vi "smartmeshIP mesh health.vi"(5 "mote and link status":T5, 11 "error in":errorcluster, 12 "mac adresses":T2) -> (2 "waveform output cluster":T1, 4 "Mote Status":T4(array[cluster]) {"mote state" items=["Lost"=0, "Negotiating"=1, "Operational"=4]}, 6 "Primary link status":T3(array[cluster]), 10 "last packet type dust":i32[](array[numeric]), 14 "Online":bool[](array[boolean]), 15 "error out":errorcluster)   [LabVIEW 2017]
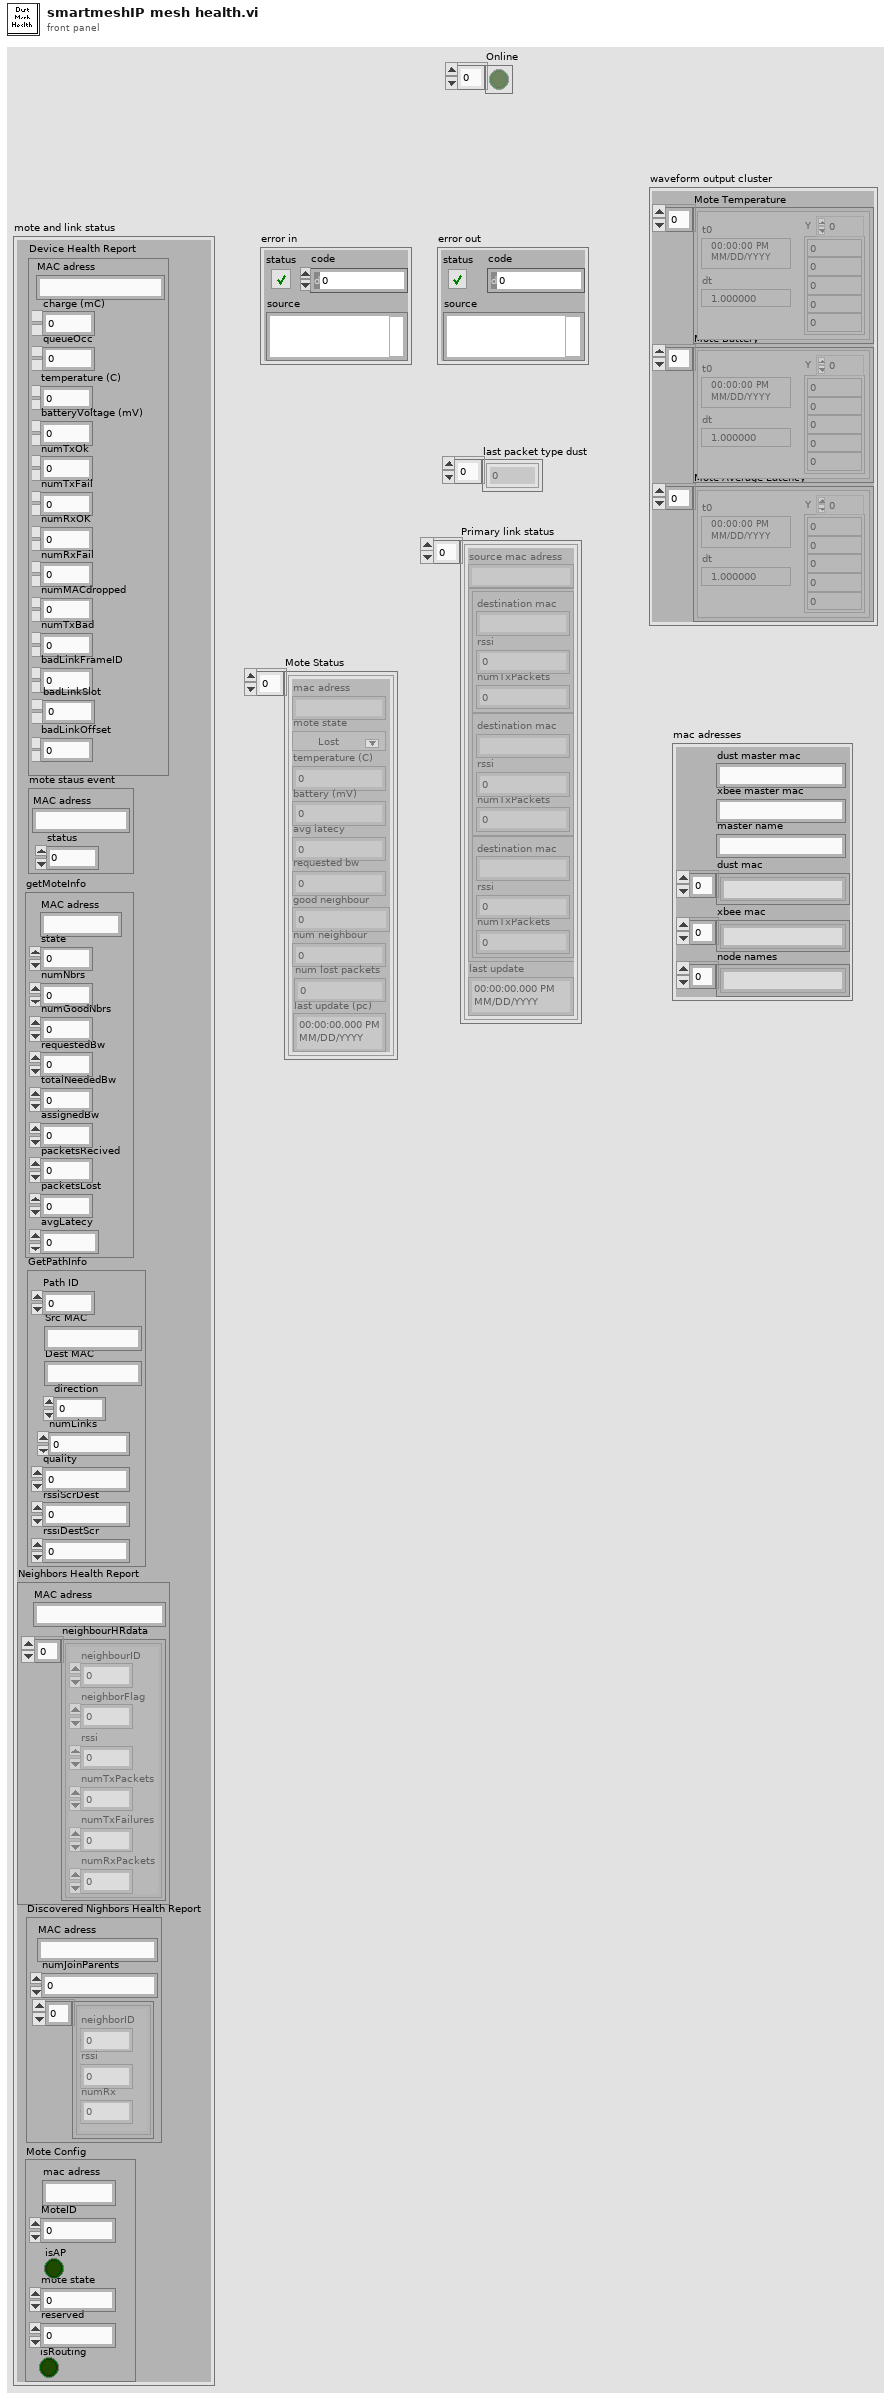
[diagram p1: front panel]
types:
  T1 = cluster{"Mote Temperature":waveform(i32)[], "Mote Battery":waveform(i32)[], "Mote Average Latency":waveform(i32)[]}
  T2 = cluster{"dust master mac":string, "xbee master mac":string, "master name":string, "dust mac":string[], "xbee mac":string[], "node names":string[]}
  T3 = cluster{"source mac adress":string, cluster{"destination mac":string, "rssi":i8, "numTxPackets":u16}[], "last update":timestamp}[]
  T4 = cluster{"mac adress":string, "mote state":u8, "temperature (C)":i8, "battery (mV)":u16, "avg latecy":u32, "requested bw":u32, "good neighbour":u8, "num neighbour":u8, "num lost packets":u8, "last update (pc)":timestamp}[]
  T5 = cluster{"Device Health Report":cluster{"MAC adress":string, "charge (mC)":u32, "queueOcc":u8, "temperature (C)":i8, "batteryVoltage (mV)":u16, "numTxOk":u16, "numTxFail":u16, "numRxOK":u16, "numRxFail":u16, "numMACdropped":u8, "numTxBad":u8, "badLinkFrameID":u8, "badLinkSlot":u32, "badLinkOffset":u8}, "mote staus event":cluster{"MAC adress":string, "status":u8}, "getMoteInfo":cluster{"MAC adress":string, "state":u8, "numNbrs":u8, "numGoodNbrs":u8, "requestedBw":u32, "totalNeededBw":u32, "assignedBw":u32, "packetsRecived":u32, "packetsLost":u32, "avgLatecy":u32}, "GetPathInfo":cluster{"Path ID":u8, "Src MAC":string, "Dest MAC":string, "direction":u8, "numLinks":u8, "quality":u8, "rssiScrDest":i8, "rssiDestScr":i8}, "Neighbors Health Report":cluster{"MAC adress":string, "neighbourHRdata":cluster{"neighbourID":u16, "neighborFlag":u8, "rssi":i8, "numTxPackets":u16, "numTxFailures":u16, "numRxPackets":u16}[]}, "Discovered Nighbors Health Report":cluster{"MAC adress":string, "numJoinParents":u8, cluster{"neighborID":u16, "rssi":i8, "numRx":u8}[]}, "Mote Config":cluster{"mac adress":string, "MoteID":u16, "isAP":bool, "mote state":u8, "reserved":u8, "isRouting":bool}}
  T6 = cluster{"MAC adress":string, "charge (mC)":u32, "queueOcc":u8, "temperature (C)":i8, "batteryVoltage (mV)":u16, "numTxOk":u16, "numTxFail":u16, "numRxOK":u16, "numRxFail":u16, "numMACdropped":u8, "numTxBad":u8, "badLinkFrameID":u8, "badLinkSlot":u32, "badLinkOffset":u8}
  T7 = cluster{"MAC adress":string, "neighbourHRdata":cluster{"neighbourID":u16, "neighborFlag":u8, "rssi":i8, "numTxPackets":u16, "numTxFailures":u16, "numRxPackets":u16}[]}
  T8 = cluster{"MAC adress":string, "state":u8, "numNbrs":u8, "numGoodNbrs":u8, "requestedBw":u32, "totalNeededBw":u32, "assignedBw":u32, "packetsRecived":u32, "packetsLost":u32, "avgLatecy":u32}
  T9 = cluster{"mac adress":string, "MoteID":u16, "isAP":bool, "mote state":u8, "reserved":u8, "isRouting":bool}
  T10 = cluster{"mac adress":string, "rssi":u8, "numTxPackets":i8}
  T11 = cluster{"time string 2":string, "mote state":u8, "temperature (C)":i8, "state":u16, "avgLatecy":u32, "avgLatecy 2":u32, "numTxBad":u8, "numTxBad 2":u8, "numTxBad 3":u8, "time string":timestamp}
  T12 = cluster{"mac adress":string, "rssi":u8, "numTxPackets":i8}[][]
  T13 = cluster{"time string 2":string, "mote state":u8, "temperature (C)":i8, "state":u16, "avgLatecy":u32, "avgLatecy 2":u32, "numTxBad":u8, "numTxBad 2":u8, "numTxBad 3":u8, "time string":timestamp}[]
  T14 = cluster{"neighbourID":u16, "neighborFlag":u8, "rssi":i8, "numTxPackets":u16, "numTxFailures":u16, "numRxPackets":u16}[]
  T15 = cluster{"mac adress":string, cluster{"Dest MAC":string, "rssi":u8, "numTxPackets":u16}[], "seconds since 1Jan1904":timestamp}
  T16 = cluster{waveform(i32)[], waveform(i32)[], waveform(i32)[]}
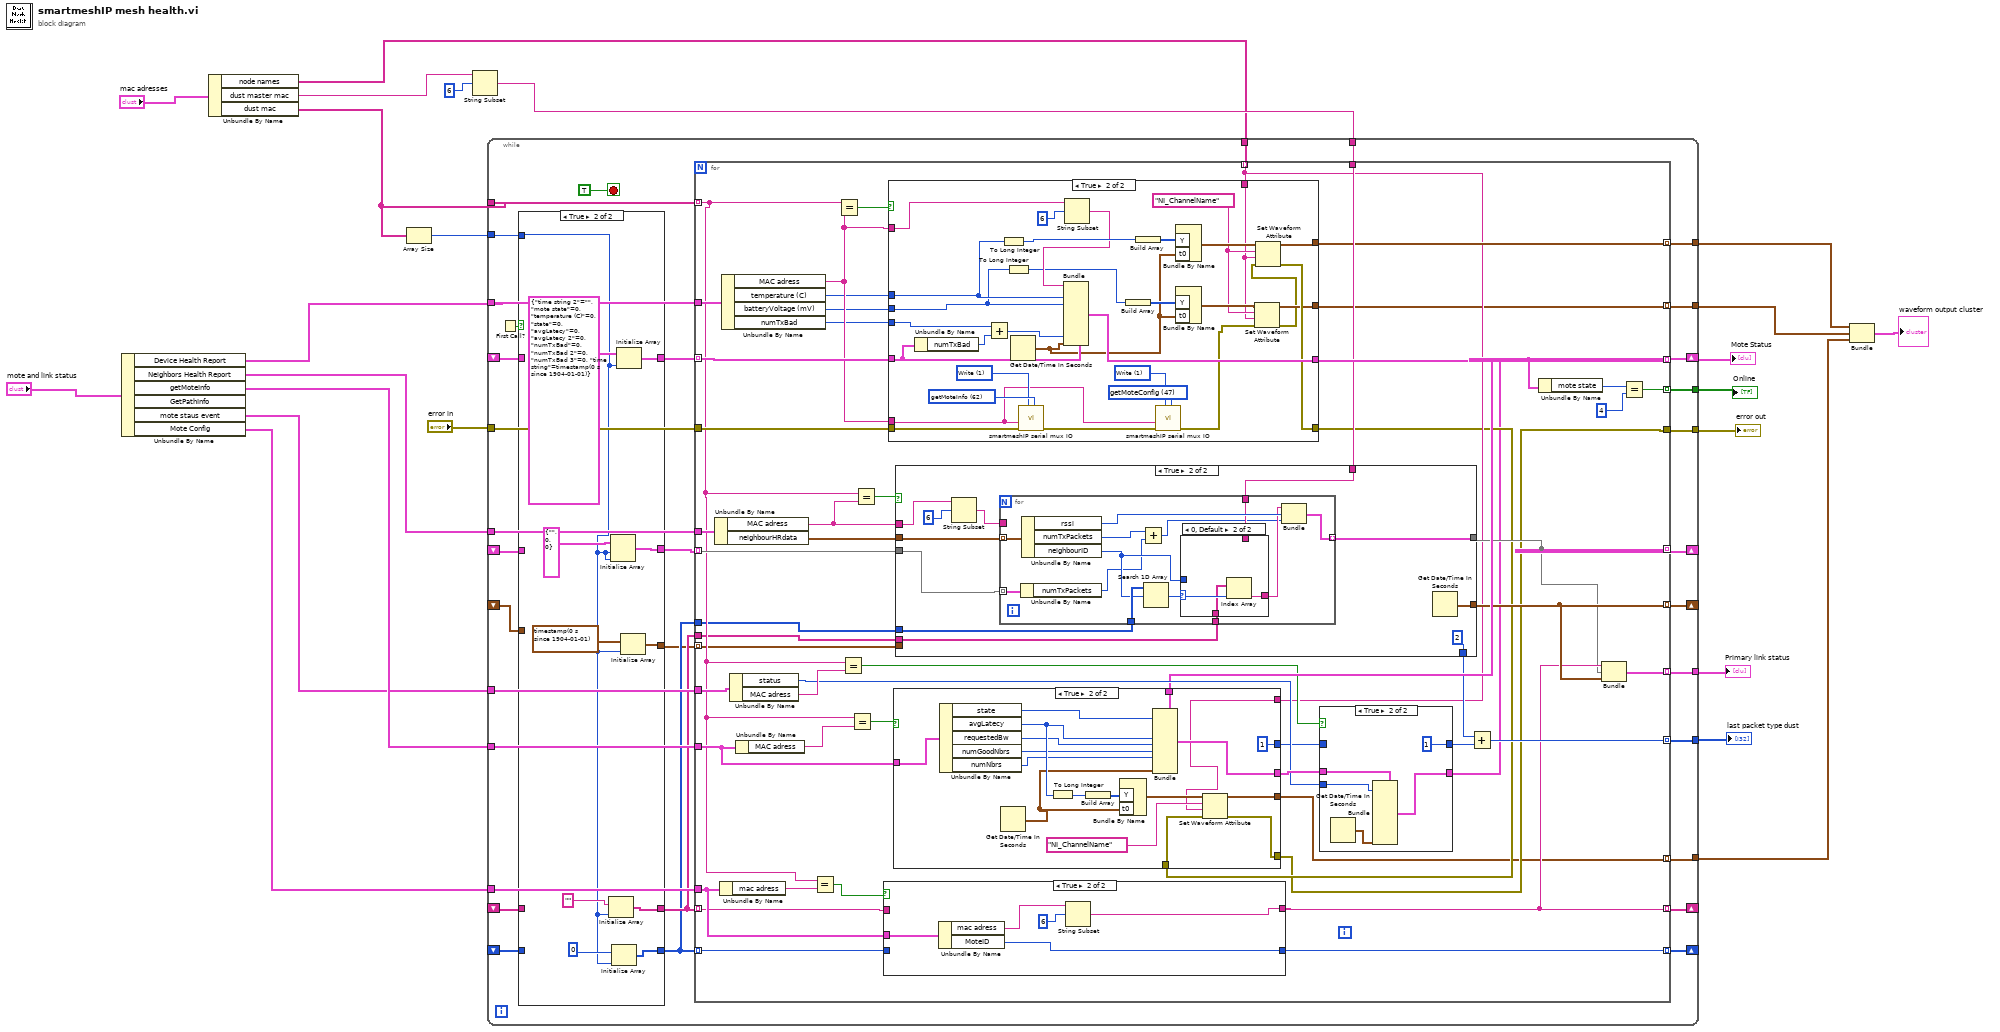
[diagram p0: block diagram]
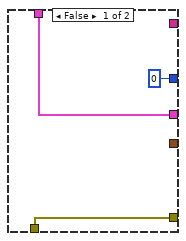
[diagram p5: hidden frame]
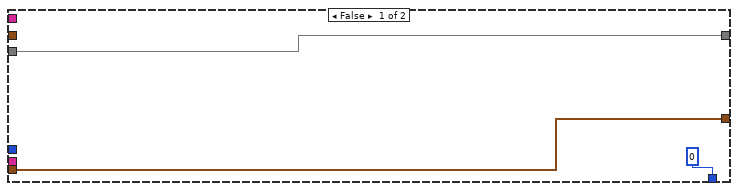
[diagram p6: hidden frame]
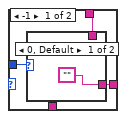
[diagram p7: hidden frame]
diagram:
  n1 = Unbundle By Name("mote and link status") -> ("Device Health Report"=w19:T6, "Neighbors Health Report"=w18:T7, "getMoteInfo"=w17:T8, "mote staus event"=w16:cluster{"MAC adress":string, "status":u8}, "Mote Config"=w15:T9)  [unwired: 1 out]
  n2 = Unbundle By Name("mac adresses") -> ("node names"=w7:string[], "dust master mac"=w8:string, "dust mac"=w9:string[])
  n3 = Array Size(array=w9) -> (size(s)=w23:i32)
  n4 = String Subset(string=w8, offset (0)=6) -> (substring=w13:string)  [unwired: 1 in]
  n5 = while {
    tunnel: w9 -> [w43]
    tunnel: w19 -> [w56]
    shift-right: [w55] -> w1
    shift-left: _ -> [w52]
    tunnel: w23 -> [w51]
    tunnel: w18 -> [w50]
    shift-right: [w47] -> _
    shift-left: _ -> [w48]
    tunnel: w17 -> [w46]
    tunnel: "error in" -> [w45]
    tunnel: [w44] -> w21
    tunnel: w16 -> [w42]
    tunnel: w15 -> [w41]
    shift-right: [w40] -> _
    shift-left: _ -> [w39]
    shift-right: [w37] -> _
    shift-left: _ -> [w36]
    shift-right: [w34] -> _
    shift-left: _ -> [w33]
    tunnel: w13 -> [w31]
    tunnel: [w30] -> w12
    tunnel: [w29] -> w11
    tunnel: [w28] -> w6
    tunnel: w7 -> [w27]
    tunnel: [w26] -> w4
    tunnel: [w25] -> w5
    tunnel: [w24] -> w2
    stop <- TRUE stop-if-true
    n6 = First Call?() -> (First Call?: T/F=w54:bool)
    n7 = case shown="True" w54 {
      tunnel: [w62 w73] -> w53
      tunnel: w52 -> [w62 _]
      tunnel: w51 -> [_ w63]
      tunnel: [w61 w72] -> w49
      tunnel: w48 -> [w61 _]
      tunnel: [w60 w69] -> w38
      tunnel: w39 -> [w60 _]
      tunnel: [w59 w66] -> w35
      tunnel: w36 -> [w59 _]
      tunnel: w33 -> [w58 _]
      tunnel: [w58 w65] -> w32
      frame False {
      }
      frame True {
        n8 = Initialize Array("" ("Dest MAC"), w63) -> (w69:string[])
        n9 = Initialize Array(T10 {"mac adress"="", "rssi"=0, "numTxPackets"=0} ("output cluster"), w63, w63) -> (w72:T12)
        n10 = Initialize Array(u16 0 ("quality"), w63) -> (w66:u16[])
        n11 = Initialize Array(T11 {"time string 2"="", "mote state"=0, "temperature (C)"=0, "state"=0, "avgLatecy"=0, "avgLatecy 2"=0, "numTxBad"=0, "numTxBad 2"=0, "numTxBad 3"=0, "time string"=timestamp(0 s since 1904-01-01)} ("output cluster"), w63) -> (w73:T13)
        n12 = Initialize Array(timestamp(0 s since 1904-01-01) ("time string"), w63) -> (w65:timestamp[])
      }
    }
    n13 = for {
      tunnel: w43 -> [w105] mode=indexing
      tunnel: w56 -> [w124]
      tunnel: [w75] -> w55 mode=indexing
      tunnel: w53 -> [w122] mode=indexing
      tunnel: w50 -> [w121]
      tunnel: [w87] -> w47 mode=indexing
      tunnel: w49 -> [w118] mode=indexing
      tunnel: w46 -> [w115]
      tunnel: w45 -> [w114]
      tunnel: [w83] -> w44
      tunnel: w42 -> [w112]
      tunnel: w41 -> [w103]
      tunnel: [w88] -> w40 mode=indexing
      tunnel: w38 -> [w102] mode=indexing
      tunnel: w38 -> [w101]
      tunnel: [w100] -> w37 mode=indexing
      tunnel: w35 -> [w99] mode=indexing
      tunnel: w35 -> [w98]
      tunnel: [w90] -> w34 mode=indexing
      tunnel: w32 -> [w97] mode=indexing
      tunnel: w31 -> [w96]
      tunnel: [w91] -> w30 mode=indexing
      tunnel: [w89] -> w29 mode=indexing
      tunnel: [w86] -> w28 mode=indexing
      tunnel: w27 -> [w85] mode=indexing
      tunnel: [w82] -> w26 mode=indexing
      tunnel: [w78] -> w25 mode=indexing
      tunnel: [w76] -> w24 mode=indexing
      n14 = Unbundle By Name(w121) -> ("MAC adress"=w107:string, "neighbourHRdata"=w119:T14)
      n15 = Unbundle By Name(w103) -> ("mac adress"=w106:string)
      n16 = Unbundle By Name(w124) -> ("MAC adress"=w109:string, "temperature (C)"=w81:i8, "batteryVoltage (mV)"=w79:u16, "numTxBad"=w80:u8)
      n17 = Unbundle By Name(w112) -> ("status"=w110:u8, "MAC adress"=w113:string)
      n18 = Unbundle By Name(w115) -> ("MAC adress"=w116:string)
      n19 = Equal?(x=w105, y=w106) -> (x = y?=w104:bool)
      n20 = Equal?(x=w105, y=w109) -> (x = y?=w123:bool)
      n21 = Equal?(x=w105, y=w113) -> (x = y?=w95:bool)
      n22 = Equal?(x=w105, y=w116) -> (x = y?=w117:bool)
      n23 = Equal?(x=w105, y=w107) -> (x = y?=w120:bool)
      n24 = case shown="True" w104 {
        tunnel: [w126 w128] -> w88
        tunnel: w103 -> [_ w131]
        tunnel: w102 -> [w126 _]
        tunnel: [w125 w127] -> w100
        tunnel: w99 -> [w125 _]
        frame False {
        }
        frame True {
          n25 = Unbundle By Name(w131) -> ("mac adress"=w129:string, "MoteID"=w127:u16)
          n26 = String Subset(string=w129, offset (0)=6) -> (substring=w128:string)  [unwired: 1 in]
        }
      }
      n27 = case shown="True" w123 {
        tunnel: w81 -> [_ w209]
        tunnel: [w196 w212] -> w108
        tunnel: w122 -> [w196 w218]
        tunnel: w109 -> [_ w219]
        tunnel: [w195 w211] -> w84
        tunnel: w114 -> [w195 w225]
        tunnel: w109 -> [_ w223]
        tunnel: w80 -> [_ w216]
        tunnel: [_ w214] -> w86
        tunnel: w85 -> [_ w201]
        tunnel: w79 -> [_ w199]
        tunnel: [_ w205] -> w78
        frame False {
        }
        frame True {
          w202 = "NI_ChannelName" ("name")
          w222 = u16 1 items=["Connect", "Write", "Read", "Close"] ("State")
          w221 = u8 47 items=["subscribe"=22, "startNetwork"=45, "setUser"=58, "setTime"=54, "setNetworkConfig"=26, "setLicense"=56, "setIPConfig"=68, "setDownstreamFrameMode"=51, "setCommonJoinKey"=66, "setAdvertising"=50, "setACLEntry"=39, "sendIP"=59, "sendData"=44, "restorFactoryDefaults"=61, "reset"=21, "radiotestTx"=35, "radiotestRx"=37, "pingMote"=42, "getTime"=23, "getSystemInfo"=46, "radiotestStatistics"=38, "getPathInfo"=48, "getNextPath"=49, "getNextACLEntry"=40, "getNetworkInfo"=64, "getNetworkConfig"=63, "getMoteLinks"=70, "getMoteInfo"=62, "getMoteConfigByld"=65, "getMoteConfig"=47, "getManagerStatistics"=53, "getLog"=43, "getLicense"=55, "getIPConfig"=67, "exchangeNetworkID"=34, "exchangeMoteJoinKey"=33, "deleteMote"=69, "deleteACLEntry"=41, "clearStatistics"=31] ("commandType_write")
          w226 = u16 1 items=["Connect", "Write", "Read", "Close"] ("State")
          w227 = u8 62 items=["subscribe"=22, "startNetwork"=45, "setUser"=58, "setTime"=54, "setNetworkConfig"=26, "setLicense"=56, "setIPConfig"=68, "setDownstreamFrameMode"=51, "setCommonJoinKey"=66, "setAdvertising"=50, "setACLEntry"=39, "sendIP"=59, "sendData"=44, "restorFactoryDefaults"=61, "reset"=21, "radiotestTx"=35, "radiotestRx"=37, "pingMote"=42, "getTime"=23, "getSystemInfo"=46, "radiotestStatistics"=38, "getPathInfo"=48, "getNextPath"=49, "getNextACLEntry"=40, "getNetworkInfo"=64, "getNetworkConfig"=63, "getMoteLinks"=70, "getMoteInfo"=62, "getMoteConfigByld"=65, "getMoteConfig"=47, "getManagerStatistics"=53, "getLog"=43, "getLicense"=55, "getIPConfig"=67, "exchangeNetworkID"=34, "exchangeMoteJoinKey"=33, "deleteMote"=69, "deleteACLEntry"=41, "clearStatistics"=31] ("commandType_write")
          n28 = Unbundle By Name(w218) -> ("numTxBad"=w217:u8)
          n29 = Add(x=w216, y=w217) -> (x+y=w207:u8)
          n30 = To Long Integer(number=w209) -> (32bit integer=w210:i32)
          n31 = To Long Integer(number=w199) -> (32bit integer=w198:i32)
          n32 = Get Date/Time In Seconds() -> (seconds since 1Jan1904=w197:timestamp)
          n33 = call "smartmeshIP serial mux IO.vi"("tx_commandType"=w227, "State"=w226, "error in"=w225, "MAC source"=w219) -> ("error out"=w220:errorcluster)  [unwired: 2 in, 5 out]
          n34 = String Subset(string=w223, offset (0)=6) -> (substring=w208:string)  [unwired: 1 in]
          n35 = Bundle(cluster=w218, "time string 2"=w208, "temperature (C)"=w209, "state"=w199, "numTxBad 3"=w207, "time string"=w197) -> (w212:T11)  [unwired: 5 in]
          n36 = Build Array(w198) -> (w200:i32[])
          n37 = Build Array(w210) -> (w215:i32[])
          n38 = call "smartmeshIP serial mux IO.vi"("tx_commandType"=w221, "State"=w222, "error in"=w220, "MAC source"=w219) -> ("error out"=w204:errorcluster)  [unwired: 2 in, 5 out]
          n39 = Bundle By Name("Y"=w215, "t0"=w197) -> (w213:waveform(i32))  [unwired: 1 in]
          n40 = Bundle By Name("Y"=w200, "t0"=w197) -> (w206:waveform(i32))  [unwired: 1 in]
          n41 = Set Waveform Attribute(4:w204, 5:w201, 6:w202, 7:w206) -> (0:w203:errorcluster, 3:w205:waveform(i32))  [unwired: 1 out]
          n42 = Set Waveform Attribute(4:w203, 5:w201, 6:w202, 7:w213) -> (0:w211:errorcluster, 3:w214:waveform(i32))  [unwired: 1 out]
        }
      }
      n43 = case shown="True" w117 {
        tunnel: w115 -> [_ w159]
        tunnel: [w141 w158] -> w111
        tunnel: w108 -> [w141 w157]
        tunnel: [0 1] -> w94
        tunnel: w85 -> [_ w152]
        tunnel: w84 -> [w139 w151]
        tunnel: [w139 w149] -> w83
        tunnel: [_ w150] -> w82
        frame False {
        }
        frame True {
          n44 = Unbundle By Name(w159) -> ("state"=w147:u8, "avgLatecy"=w146:u32, "requestedBw"=w145:u32, "numGoodNbrs"=w144:u8, "numNbrs"=w143:u8)
          n45 = Get Date/Time In Seconds() -> (seconds since 1Jan1904=w142:timestamp)
          n46 = To Long Integer(number=w146) -> (32bit integer=w148:i32)
          n47 = Build Array(w148) -> (w155:i32[])
          n48 = Bundle By Name("Y"=w155, "t0"=w142) -> (w154:waveform(i32))  [unwired: 1 in]
          n49 = Bundle(cluster=w157, "mote state"=w147, "avgLatecy"=w146, "avgLatecy 2"=w145, "numTxBad"=w144, "numTxBad 2"=w143, "time string"=w142) -> (w158:T11)  [unwired: 4 in]
          n50 = Set Waveform Attribute(4:w151, 5:w152, 6:"NI_ChannelName" ("name"), 7:w154) -> (0:w149:errorcluster, 3:w150:waveform(i32))  [unwired: 1 out]
        }
      }
      n51 = case shown="True" w120 {
        tunnel: w119 -> [_ w173]
        tunnel: [w162 w163] -> w87
        tunnel: w118 -> [w162 w165]
        tunnel: w107 -> [_ w171]
        tunnel: w101 -> [_ w168]
        tunnel: w98 -> [_ w169]
        tunnel: [w161 w167] -> w90
        tunnel: w97 -> [w161 _]
        tunnel: w96 -> [_ w166]
        tunnel: [0 2] -> w92
        frame False {
        }
        frame True {
          n52 = String Subset(string=w171, offset (0)=6) -> (substring=w170:string)  [unwired: 1 in]
          n53 = for {
            tunnel: w173 -> [w186] mode=indexing
            tunnel: [w185] -> w163 mode=indexing
            tunnel: w170 -> [_]
            tunnel: w169 -> [w183]
            tunnel: w168 -> [w182]
            tunnel: w166 -> [w181]
            tunnel: w165 -> [w178] mode=indexing
            n54 = Unbundle By Name(w178) -> ("numTxPackets"=w176:u16)
            n55 = Unbundle By Name(w186) -> ("rssi"=w184:i8, "numTxPackets"=w177:u16, "neighbourID"=w179:u16)
            n56 = Add(x=w177, y=w176) -> (x+y=w174:u16)
            n57 = Search 1D Array(1D array=w183, element=w179) -> (index of element=w180:i32)  [unwired: 1 in]
            n58 = case shown="0, Default" w180 {
              selector: w180 -> [_ w194]
              tunnel: w182 -> [_ w193]
              tunnel: [w189 w192] -> w175
              tunnel: w181 -> [w188 _]
              tunnel: w179 -> [w187 _]
              frame -1 {
                n59 = case shown="0, Default" w187 {
                  tunnel: ["" ("Dest MAC") w191] -> w189
                  tunnel: w188 -> [_ w191]
                  frame 0, Default {
                  }
                  frame 1 {
                  }
                }
              }
              frame 0, Default {
                n60 = Index Array(array=w193, index=w194) -> (element=w192:string)
              }
            }
            n61 = Bundle("Dest MAC"=w175, "rssi"=w184, w174) -> (w185:cluster{"Dest MAC":string, "rssi":i8, u16})  [unwired: 1 in]
          }
          n62 = Get Date/Time In Seconds() -> (seconds since 1Jan1904=w167:timestamp)
        }
      }
      n63 = case shown="True" w95 {
        tunnel: w111 -> [w133 w138]
        tunnel: [w133 w137] -> w75
        tunnel: w110 -> [_ w134]
        tunnel: w94 -> [w132 _]
        tunnel: [w132 1] -> w93
        frame False {
        }
        frame True {
          n64 = Get Date/Time In Seconds() -> (seconds since 1Jan1904=w135:timestamp)
          n65 = Bundle(cluster=w138, "mote state"=w134, "time string"=w135) -> (w137:T11)  [unwired: 8 in]
        }
      }
      n66 = Add(x=w92, y=w93) -> (x+y=w91:i32)
      n67 = Unbundle By Name(w75) -> ("mote state"=w74:u8)
      n68 = Bundle("mac adress"=w88, w87, "seconds since 1Jan1904"=w90) -> (w89:T15)  [unwired: 1 in]
      n69 = Equal?(x=w74, y=u8 4) -> (x = y?=w76:bool)
    }
  }
  "error out" <- w21
  "Mote Status" <- w1
  "last packet type dust" <- w12
  "Primary link status" <- w11
  "Online" <- w2
  n70 = Bundle(w6, w5, w4) -> (→"waveform output cluster":T16)  [unwired: 1 in]
